vi "ItemSelected.vi"(8 "error in (no error)":errorcluster, 9 "Siblings":refnum<data-value>[](array[refnum]), 10 "MenuItem in":refnum<class "MGI_MenuItem.lvclass">, 11 "MGI_ToggleText in":refnum<class "MGI_ToggleText.lvclass">) -> (0 "error out":errorcluster, 2 "MenuItem out":refnum<class "MGI_MenuItem.lvclass">, 3 "MGI_ToggleText out":refnum<class "MGI_ToggleText.lvclass">)   [LabVIEW 2016, in "MGI_ToggleText.lvclass"]
doc: "Toggles the the text\n\nAuthored by Derek E. Trepanier\nsupport@mooregoodideas.com\nwww.mooregoodideas.com\n\nCopyright (c) 2012, Moore Good Ideas, Inc.\n\nAll rights reserved.\n\nRedistribution and use in source and binary forms, with or without modification, are permitted provided that the following conditions are met:\n\n * Redistributions of source code must retain the above copyright notice, this list of conditions and the following disclaimer.\n * Redistributions in binary form must reproduce the above copyright notice, this list of conditions and the following disclaimer in the documentation and/or other materials provided with the distribution.\n * Neither the name of Moore Good Ideas, Inc. nor the names of its contributors may be used to endorse or promote products derived from this software without specific prior written permission.\n\nTHIS SOFTWARE IS PROVIDED BY THE COPYRIGHT HOLDERS AND CONTRIBUTORS \"AS IS\" AND ANY EXPRESS OR IMPLIED WARRANTIES, INCLUDING, BUT NOT LIMITED TO, THE IMPLIED WARRANTIES OF MERCHANTABILITY AND FITNESS FOR A PARTICULAR PURPOSE ARE DISCLAIMED. IN NO EVENT SHALL THE COPYRIGHT OWNER OR CONTRIBUTORS BE LIABLE FOR ANY DIRECT, INDIRECT, INCIDENTAL, SPECIAL, EXEMPLARY, OR CONSEQUENTIAL DAMAGES (INCLUDING, BUT NOT LIMITED TO, PROCUREMENT OF SUBSTITUTE GOODS OR SERVICES; LOSS OF USE, DATA, OR PROFITS; OR BUSINESS INTERRUPTION) HOWEVER CAUSED AND ON ANY THEORY OF LIABILITY, WHETHER IN CONTRACT, STRICT LIABILITY, OR TORT (INCLUDING NEGLIGENCE OR OTHERWISE) ARISING IN ANY WAY OUT OF THE USE OF THIS SOFTWARE, EVEN IF ADVISED OF THE POSSIBILITY OF SUCH DAMAGE."
uses:
  <userlib>/_MGI/Menu Building/SelectionType/ToggleText/MGI_ToggleText.lvclass
  <userlib>/_MGI/Menu Building/MenuItem/MGI_MenuItem.lvclass
  <userlib>/_MGI/Menu Building/SelectionType/ToggleText/MGI_ToggleText.lvclass/MGI_ToggleText.ctl
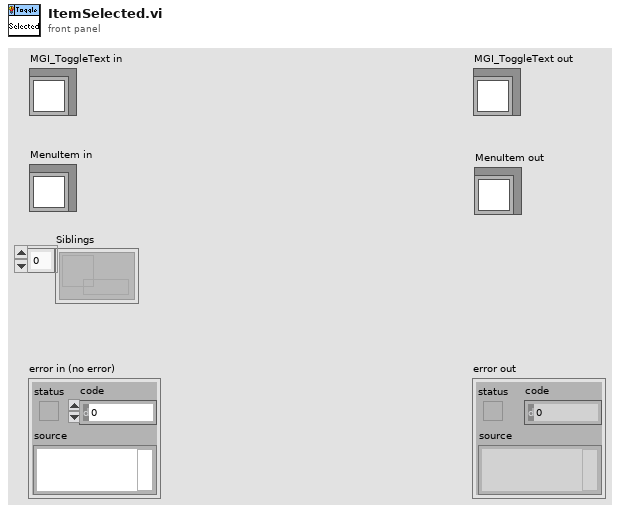
[diagram p1: front panel]
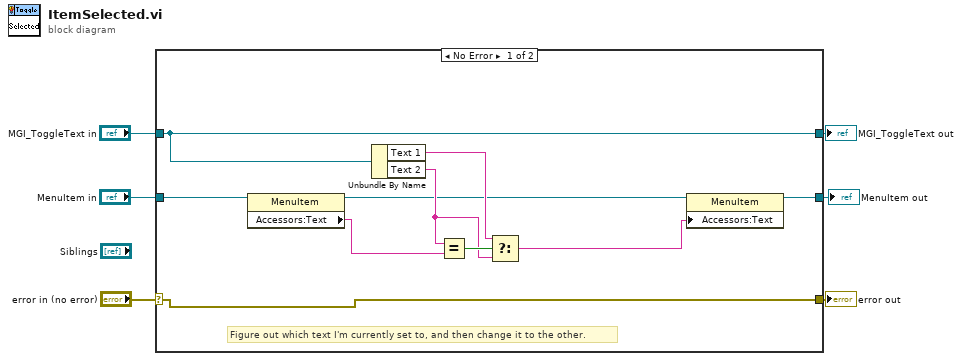
[diagram p0: block diagram]
diagram:
  n1 = case shown="No Error" "error in (no error)" {
    selector: "error in (no error)" -> [w12 w19]
    tunnel: [w12 w19] -> w5
    tunnel: [w16 w18] -> w4
    tunnel: "MGI_ToggleText in" -> [w16 w18]
    tunnel: "MenuItem in" -> [w9 w17]
    tunnel: [w11 w17] -> w1
    frame No Error {
      # "Figure out which text I'm currently set to, and then change it to the other."
      n2 = property class="MenuItem"(reference=w9) -> (reference out=w8:refnum<class "MGI_MenuItem.lvclass">, "Accessors:Text"=w7:string)  [unwired: 1 in, 1 out]
      n3 = Unbundle By Name(w16) -> ("Text 1"=w14:string, "Text 2"=w13:string)
      n4 = Equal?(x=w13, y=w7) -> (x = y?=w15:bool)
      n5 = Select(t=w14, s=w15, f=w13) -> (s? t:f=w10:string)
      n6 = property class="MenuItem"(reference=w8, "Accessors:Text"=w10) -> (reference out=w11:refnum<class "MGI_MenuItem.lvclass">)  [unwired: 1 in, 1 out]
    }
    frame Error {
    }
  }
  "error out" <- w5
  "MGI_ToggleText out" <- w4
  "MenuItem out" <- w1
